vi "Get_Variant_Cluster_Element_by_Name.vi"(8 "error in (no error)":errorcluster, 10 "Element name":string, 11 "Cluster":variant) -> (0 "error out":errorcluster, 2 "Found?":bool, 3 "VElement":variant)   [LabVIEW 2012]
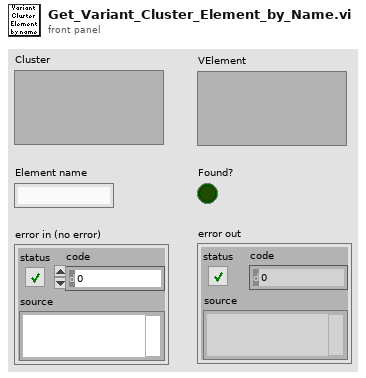
[diagram p1: front panel]
types:
  T1 = cluster{"length":u16, "private":u8, "type":enum8{"<Null>", "I8", "I16", "I32", "I64", "U8", "U16", "U32", "U64", "SGL", "DBL", "EXT", "CSG", "CDB", "CXT", "0x0F", "0x10", "0x11", "0x12", "0x13", "0x14", "Enum U8", "Enum U16", "Enum U32", "Enum U64", "SGL PQ", "DBL PQ", "EXT PQ", "CSG PQ", "CDB PQ", "CXT PQ", "0x1F", "0x20", "Boolean", "0x22", "0x23", "0x24", "0x25", "0x26", "0x27", "0x28", "0x29", "0x2A", "0x2B", "0x2C", "0x2D", "0x2E", "0x2F", "String", "0x31", "Path", "Pict", "0x34", "0x35", "0x36", "DAQ", "0x38", "0x39", "0x3A", "0x3B", "0x3C", "0x3D", "0x3E", "0x3F", "Array", "0x41", "0x42", "0x43", "0x44", "0x45", "0x46", "0x47", "0x48", "0x49", "0x4A", "0x4B", "0x4C", "0x4D", "0x4E", "0x4F", "Cluster", "0x51", "0x52", "Variant", "Waveform", "0x55", "0x56", "0x57", "0x58", "0x59", "0x5A", "0x5B", "0x5C", "0x5D", "0x5E", "0x5F", "0x60", "0x61", "0x62", "0x63", "0x64", "0x65", "0x66", "0x67", "0x68", "0x69", "0x6A", "0x6B", "0x6C", "0x6D", "0x6E", "0x6F", "Refnum"}, "# elements":u16}
  T2 = enum8{"<Null>", "I8", "I16", "I32", "I64", "U8", "U16", "U32", "U64", "SGL", "DBL", "EXT", "CSG", "CDB", "CXT", "0x0F", "0x10", "0x11", "0x12", "0x13", "0x14", "Enum U8", "Enum U16", "Enum U32", "Enum U64", "SGL PQ", "DBL PQ", "EXT PQ", "CSG PQ", "CDB PQ", "CXT PQ", "0x1F", "0x20", "Boolean", "0x22", "0x23", "0x24", "0x25", "0x26", "0x27", "0x28", "0x29", "0x2A", "0x2B", "0x2C", "0x2D", "0x2E", "0x2F", "String", "0x31", "Path", "Pict", "0x34", "0x35", "0x36", "DAQ", "0x38", "0x39", "0x3A", "0x3B", "0x3C", "0x3D", "0x3E", "0x3F", "Array", "0x41", "0x42", "0x43", "0x44", "0x45", "0x46", "0x47", "0x48", "0x49", "0x4A", "0x4B", "0x4C", "0x4D", "0x4E", "0x4F", "Cluster", "0x51", "0x52", "Variant", "Waveform", "0x55", "0x56", "0x57", "0x58", "0x59", "0x5A", "0x5B", "0x5C", "0x5D", "0x5E", "0x5F", "0x60", "0x61", "0x62", "0x63", "0x64", "0x65", "0x66", "0x67", "0x68", "0x69", "0x6A", "0x6B", "0x6C", "0x6D", "0x6E", "0x6F", "Refnum"}
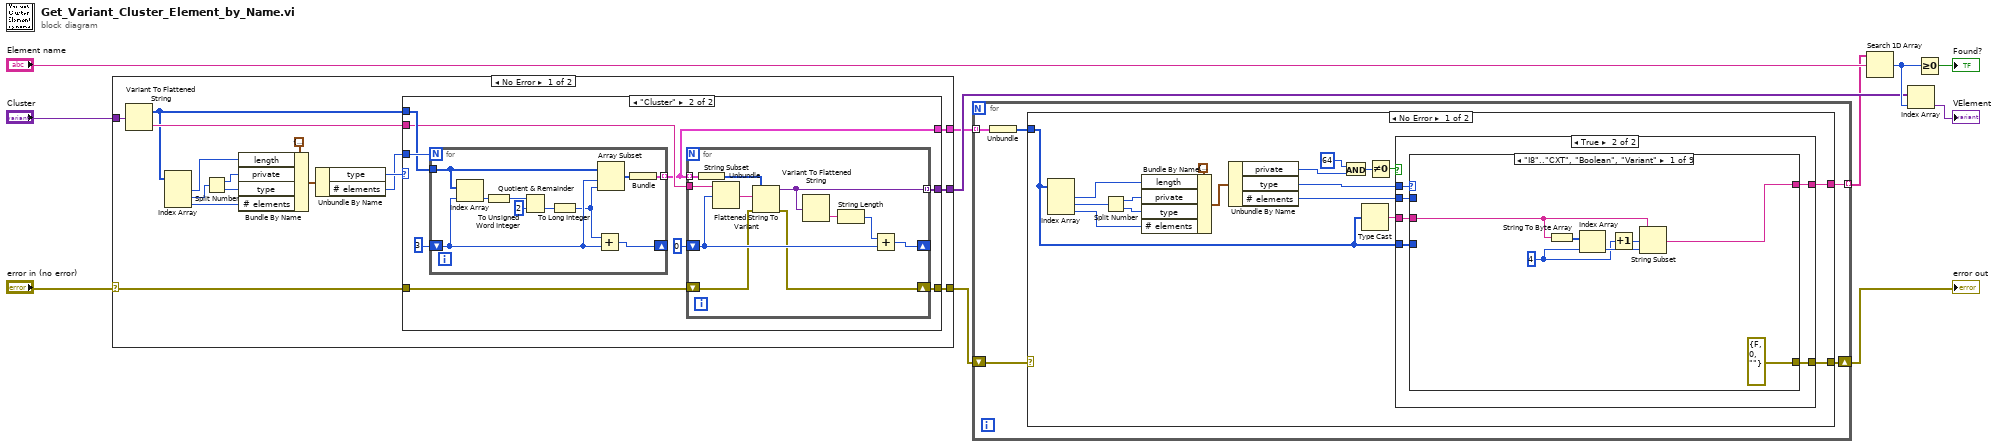
[diagram p0: block diagram]
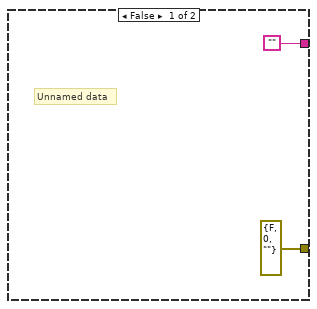
[diagram p2: hidden frame]
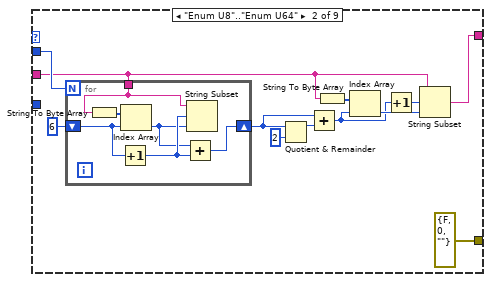
[diagram p3: hidden frame]
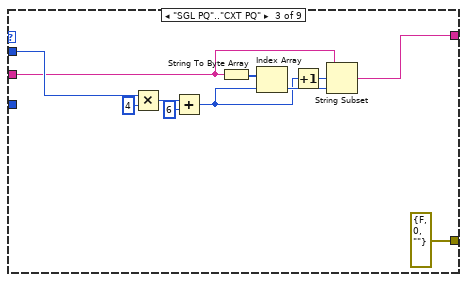
[diagram p4: hidden frame]
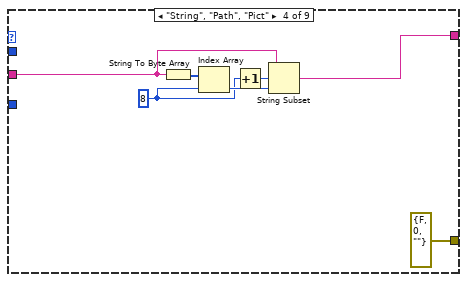
[diagram p5: hidden frame]
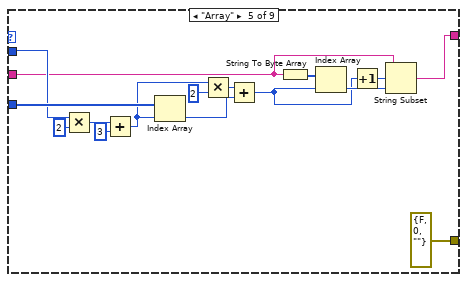
[diagram p6: hidden frame]
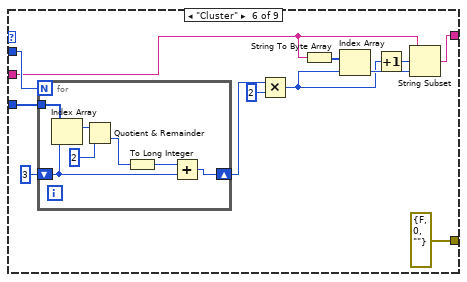
[diagram p7: hidden frame]
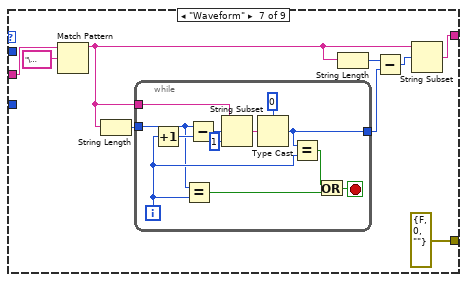
[diagram p8: hidden frame]
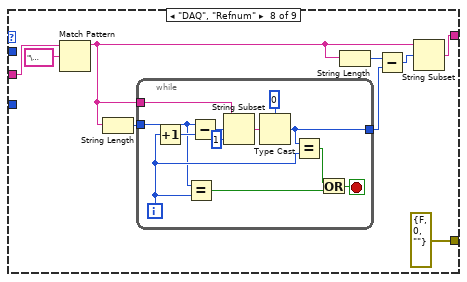
[diagram p9: hidden frame]
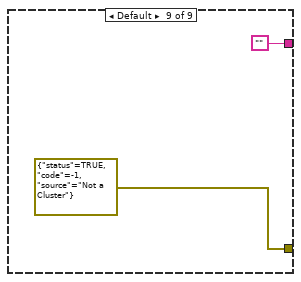
[diagram p10: hidden frame]
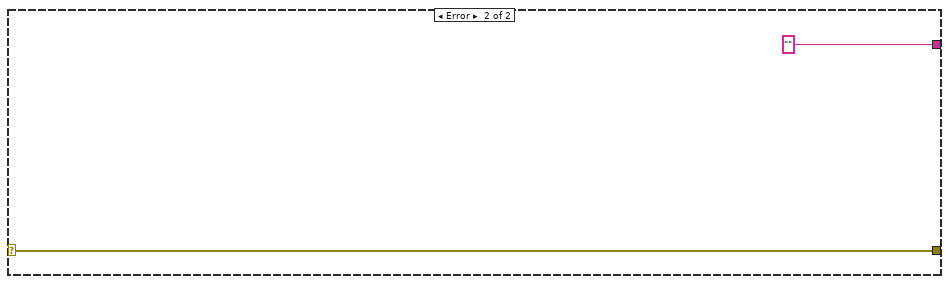
[diagram p11: hidden frame]
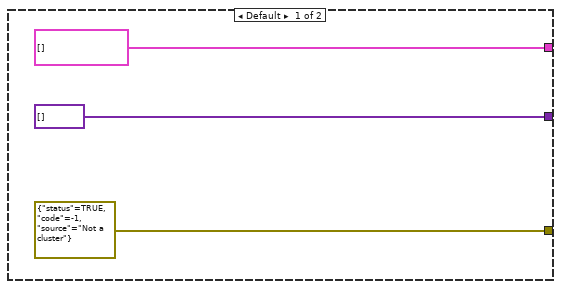
[diagram p12: hidden frame]
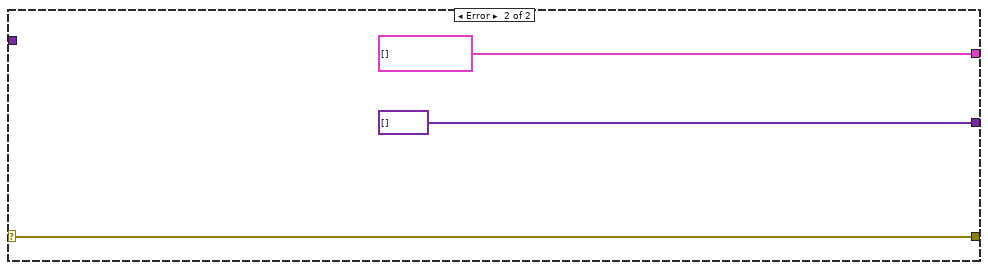
[diagram p13: hidden frame]
diagram:
  n1 = case shown="No Error" "error in (no error)" {
    selector: "error in (no error)" -> [w14 w63]
    tunnel: [w27 w63] -> w1
    tunnel: [w25 variant[] []] -> w6
    tunnel: "Cluster" -> [w24 _]
    tunnel: [w13 cluster{i16[]}[] []] -> w3
    frame No Error {
      n2 = Variant To Flattened String(Variant=w24) -> (data string=w23:string, 1:w17:i16[])
      n3 = Index Array(array=w17) -> (element #1=w18:i16, element #2=w21:i16, element #3=w22:i16)  [unwired: 3 in]
      n4 = Split Number(x=w21) -> (hi(x)=w19:u8, lo(x)=w20:u8)
      n5 = Bundle By Name(cluster=T1 {"length"=0, "private"=0, "type"=enum."<Null>", "# elements"=0} ("Type Descriptor Header"), "length"=w18, "private"=w19, "type"=w20, "# elements"=w22) -> (w16:T1)
      n6 = Unbundle By Name(w16) -> ("type"=w26:T2, "# elements"=w15:u16)
      n7 = case shown="\"Cluster\"" w26 {
        tunnel: [errorcluster {"status"=TRUE, "code"=-1, "source"="Not a cluster"} ("error out") w34] -> w27
        tunnel: [variant[] [] w35] -> w25
        tunnel: w17 -> [_ w37]
        tunnel: w23 -> [_ w36]
        tunnel: w15 -> [_ w38]
        tunnel: w14 -> [_ w33]
        tunnel: [cluster{i16[]}[] [] w32] -> w13
        frame Default {
        }
        frame "Cluster" {
          n8 = for {
            N: w38 -> [_]
            shift-right: [w58] -> _
            shift-left: 3 -> [w57]
            tunnel: w37 -> [w59]
            tunnel: [w53] -> w32 mode=indexing
            n9 = Index Array(array=w59, index=w57) -> (element=w55:i16)
            n10 = To Unsigned Word Integer(number=w55) -> (unsigned 16bit integer=w52:u16)
            n11 = Quotient & Remainder(x=w52, y=u16 2) -> (floor(x/y)=w56:u16)  [unwired: 1 out]
            n12 = To Long Integer(number=w56) -> (32bit integer=w51:i32)
            n13 = Add(x=w51, y=w57) -> (x+y=w58:i32)
            n14 = Array Subset(array=w59, index=w57, length=w51) -> (w60:i16[])
            n15 = Bundle(w60) -> (w53:cluster{i16[]})  [unwired: 1 in]
          }
          n16 = for {
            tunnel: w36 -> [w47]
            tunnel: [w50] -> w35 mode=indexing
            shift-right: [w44] -> _
            shift-left: 0 -> [w46]
            shift-right: [w42] -> w34
            shift-left: w33 -> [w43]
            tunnel: w32 -> [w41] mode=indexing
            n17 = Unbundle(w41) -> (w40:i16[])
            n18 = String Subset(string=w47, offset (0)=w46) -> (substring=w48:string)  [unwired: 1 in]
            n19 = Flattened String To Variant(4:w43, 6:w48, 7:w40) -> (0:w42:errorcluster, 3:w50:variant)
            n20 = Variant To Flattened String(Variant=w50) -> (data string=w49:string)  [unwired: 1 out]
            n21 = String Length(string=w49) -> (length=w45:i32)
            n22 = Add(x=w45, y=w46) -> (x+y=w44:i32)
          }
        }
      }
    }
    frame Error {
    }
  }
  n23 = for {
    tunnel: w3 -> [w68] mode=indexing
    shift-right: [w65] -> w5
    shift-left: w1 -> [w66]
    tunnel: [w64] -> w4 mode=indexing
    n24 = Unbundle(w68) -> (w67:i16[])
    n25 = case shown="No Error" w66 {
      selector: w66 -> [_ w217]
      tunnel: w67 -> [w71 _]
      tunnel: [w83 "" ("Last PString")] -> w64
      tunnel: [w77 w217] -> w65
      frame No Error {
        n26 = Index Array(array=w71) -> (element #1=w72:i16, element #2=w75:i16, element #3=w76:i16)  [unwired: 3 in]
        n27 = Split Number(x=w75) -> (hi(x)=w73:u8, lo(x)=w74:u8)
        n28 = Bundle By Name(cluster=T1 {"length"=0, "private"=0, "type"=enum."<Null>", "# elements"=0} ("Type Descriptor Header"), "length"=w72, "private"=w73, "type"=w74, "# elements"=w76) -> (w70:T1)
        n29 = Unbundle By Name(w70) -> ("private"=w79:u8, "type"=w78:T2, "# elements"=w85:u16)
        n30 = And(x=u8 64, y=w79) -> (x .and. y?=w82:u8)
        n31 = Type Cast(x=w71) -> (*(type *) &x=w84:string)  [unwired: 1 in]
        n32 = Not Equal To 0?(x=w82) -> (x != 0?=w81:bool)
        n33 = case shown="True" w81 {
          tunnel: [errorcluster {"status"=FALSE, "code"=0, "source"=""} ("error out") w93] -> w77
          tunnel: w78 -> [_ w92]
          tunnel: w84 -> [_ w91]
          tunnel: ["" w90] -> w83
          tunnel: w85 -> [_ w89]
          tunnel: w71 -> [_ w88]
          frame False {
            # "Unnamed data"
          }
          frame True {
            n34 = case shown="\"I8\"..\"CXT\", \"Boolean\", \"Variant\"" w92 {
              tunnel: [errorcluster {"status"=FALSE, "code"=0, "source"=""} ("error out") errorcluster {"status"=FALSE, "code"=0, "source"=""} ("error out") errorcluster {"status"=FALSE, "code"=0, "source"=""} ("error out") errorcluster {"status"=FALSE, "code"=0, "source"=""} ("error out") errorcluster {"status"=FALSE, "code"=0, "source"=""} ("error out") errorcluster {"status"=FALSE, "code"=0, "source"=""} ("error out") errorcluster {"status"=FALSE, "code"=0, "source"=""} ("error out") errorcluster {"status"=FALSE, "code"=0, "source"=""} ("error out") errorcluster {"status"=TRUE, "code"=-1, "source"="Not a Cluster"} ("error out")] -> w93
              tunnel: w91 -> [w94 w102 w120 w131 w138 w155 w173 w194 _]
              tunnel: [w95 w101 w119 w130 w137 w153 w172 w193 ""] -> w90
              tunnel: w89 -> [_ w109 w128 _ w144 w163 _ _ _]
              tunnel: w88 -> [_ _ _ _ w151 w162 _ _ _]
              frame "I8".."CXT", "Boolean", "Variant" {
                w96 = 4 ("offset (0)")
                n35 = String To Byte Array(string=w94) -> (unsigned byte array=w99:u8[])
                n36 = Index Array(array=w99, index=w96) -> (element=w97:u8)
                n37 = Increment(x=w96) -> (x+1=w98:i32)
                n38 = String Subset(string=w94, offset (0)=w98, length (rest)=w97) -> (substring=w95:string)
              }
              frame "Enum U8".."Enum U64" {
                n39 = for {
                  N: w109 -> [_]
                  tunnel: w102 -> [w115]
                  shift-right: [w114] -> w111
                  shift-left: 6 -> [w113]
                  n40 = String To Byte Array(string=w115) -> (unsigned byte array=w118:u8[])
                  n41 = Increment(x=w113) -> (x+1=w117:i32)
                  n42 = Index Array(array=w118, index=w113) -> (element=w116:u8)
                  n43 = Add(x=w116, y=w117) -> (x+y=w114:i32)
                  n44 = String Subset(string=w115, offset (0)=w117, length (rest)=w116) -> ()  [unwired: 1 out]
                }
                n45 = Quotient & Remainder(x=w111, y=2) -> (x-y*floor(x/y)=w107:i32)  [unwired: 1 out]
                n46 = Add(x=w111, y=w107) -> (x+y=w103:i32)
                n47 = String To Byte Array(string=w102) -> (unsigned byte array=w106:u8[])
                n48 = Index Array(array=w106, index=w103) -> (element=w104:u8)
                n49 = Increment(x=w103) -> (x+1=w105:i32)
                n50 = String Subset(string=w102, offset (0)=w105, length (rest)=w104) -> (substring=w101:string)
              }
              frame "SGL PQ".."CXT PQ" {
                n51 = Multiply(x=w128, y=u16 4) -> (x*y=w126:u16)
                n52 = Add(x=w126, y=u16 6) -> (x+y=w121:u16)
                n53 = String To Byte Array(string=w120) -> (unsigned byte array=w122:u8[])
                n54 = Index Array(array=w122, index=w121) -> (element=w124:u8)
                n55 = Increment(x=w121) -> (x+1=w123:u16)
                n56 = String Subset(string=w120, offset (0)=w123, length (rest)=w124) -> (substring=w119:string)
              }
              frame "String", "Path", "Pict" {
                w132 = 8 ("offset (0)")
                n57 = String To Byte Array(string=w131) -> (unsigned byte array=w133:u8[])
                n58 = Index Array(array=w133, index=w132) -> (element=w135:u8)
                n59 = Increment(x=w132) -> (x+1=w134:i32)
                n60 = String Subset(string=w131, offset (0)=w134, length (rest)=w135) -> (substring=w130:string)
              }
              frame "Array" {
                n61 = Multiply(x=w144, y=u16 2) -> (x*y=w146:u16)
                n62 = Add(x=w146, y=u16 3) -> (x+y=w143:u16)
                n63 = Index Array(array=w151, index=w143) -> (element=w148:i16)
                n64 = Multiply(x=w143, y=u16 2) -> (x*y=w149:u16)
                n65 = Add(x=w149, y=w148) -> (x+y=w139:u16)
                n66 = String To Byte Array(string=w138) -> (unsigned byte array=w142:u8[])
                n67 = Index Array(array=w142, index=w139) -> (element=w140:u8)
                n68 = Increment(x=w139) -> (x+1=w141:u16)
                n69 = String Subset(string=w138, offset (0)=w141, length (rest)=w140) -> (substring=w137:string)
              }
              frame "Cluster" {
                n70 = for {
                  N: w163 -> [_]
                  shift-right: [w170] -> w160
                  shift-left: 3 -> [w169]
                  tunnel: w162 -> [w171]
                  n71 = Index Array(array=w171, index=w169) -> (element=w167:i16)
                  n72 = Quotient & Remainder(x=w167, y=i16 2) -> (floor(x/y)=w168:i16)  [unwired: 1 out]
                  n73 = To Long Integer(number=w168) -> (32bit integer=w165:i32)
                  n74 = Add(x=w165, y=w169) -> (x+y=w170:i32)
                }
                n75 = Multiply(x=w160, y=2) -> (x*y=w154:i32)
                n76 = String To Byte Array(string=w155) -> (unsigned byte array=w156:u8[])
                n77 = Index Array(array=w156, index=w154) -> (element=w158:u8)
                n78 = Increment(x=w154) -> (x+1=w157:i32)
                n79 = String Subset(string=w155, offset (0)=w157, length (rest)=w158) -> (substring=w153:string)
              }
              frame "Waveform" {
                n80 = Match Pattern(string=w173, regular expression="\u0000$" ("*(type *) &x")) -> (before substring=w175:string)  [unwired: 1 in, 3 out]
                n81 = String Length(string=w175) -> (length=w174:i32)
                n82 = while {
                  tunnel: [w187] -> w179
                  tunnel: w174 -> [w182]
                  tunnel: w175 -> [w191]
                  i -> [w185]
                  stop <- w184 stop-if-true
                  n83 = Increment(x=w185) -> (x+1=w186:i32)
                  n84 = Equal?(x=w182, y=w185) -> (x = y?=w181:bool)
                  n85 = Subtract(x=w182, y=w186) -> (x-y=w190:i32)
                  n86 = String Subset(string=w191, offset (0)=w190, length (rest)=1 ("length (rest)")) -> (substring=w189:string)
                  n87 = Type Cast(type=u8 0, x=w189) -> (*(type *) &x=w187:u8)
                  n88 = Equal?(x=w187, y=w185) -> (x = y?=w183:bool)
                  n89 = Or(x=w183, y=w181) -> (x .or. y?=w184:bool)
                }
                n90 = String Length(string=w175) -> (length=w177:i32)
                n91 = Subtract(x=w177, y=w179) -> (x-y=w178:i32)
                n92 = String Subset(string=w175, offset (0)=w178) -> (substring=w172:string)  [unwired: 1 in]
              }
              frame "DAQ", "Refnum" {
                n93 = Match Pattern(string=w194, regular expression="\u0000$" ("*(type *) &x")) -> (before substring=w199:string)  [unwired: 1 in, 3 out]
                n94 = String Length(string=w199) -> (length=w200:i32)
                n95 = while {
                  tunnel: [w208] -> w195
                  tunnel: w200 -> [w203]
                  tunnel: w199 -> [w212]
                  i -> [w206]
                  stop <- w205 stop-if-true
                  n96 = Increment(x=w206) -> (x+1=w207:i32)
                  n97 = Equal?(x=w203, y=w206) -> (x = y?=w202:bool)
                  n98 = Subtract(x=w203, y=w207) -> (x-y=w211:i32)
                  n99 = String Subset(string=w212, offset (0)=w211, length (rest)=1 ("length (rest)")) -> (substring=w210:string)
                  n100 = Type Cast(type=u8 0, x=w210) -> (*(type *) &x=w208:u8)
                  n101 = Equal?(x=w208, y=w206) -> (x = y?=w204:bool)
                  n102 = Or(x=w204, y=w202) -> (x .or. y?=w205:bool)
                }
                n103 = String Length(string=w199) -> (length=w197:i32)
                n104 = Subtract(x=w197, y=w195) -> (x-y=w196:i32)
                n105 = String Subset(string=w199, offset (0)=w196) -> (substring=w193:string)  [unwired: 1 in]
              }
              frame Default {
              }
            }
          }
        }
      }
      frame Error {
      }
    }
  }
  "error out" <- w5
  n106 = Search 1D Array(1D array=w4, element="Element name") -> (index of element=w11:i32)  [unwired: 1 in]
  n107 = Index Array(array=w6, index=w11) -> (element=→"VElement":variant)
  n108 = Greater Or Equal To 0?(x=w11) -> (x >= 0?=→"Found?":bool)
